vi "Waveform generation_dual color_plane by plane - backupCopy.vi"(0 "Number of Steps":dbl, 1 "488 LASER Intensity":dbl(slide) scale=0.0..10.0, 2 "SPIMA Obj Ampl":dbl, 3 "SPIMB Z- galvo amplitude":dbl, 4 "SPIMA Z-Galvo Offset":dbl(slide) scale=0.0..10.0, 5 "SPIMA Z-Galvo Amplitude":dbl(slide) scale=0.0..10.0, 6 "SPIMA Camera trigger":dbl, 7 "SPIMA Obejective Offset":dbl(slide) scale=0.0..10.0, 8 "SPIMB Obejective Offset":dbl(slide) scale=0.0..10.0, 9 "SPIMA Y-Galvo Offset":dbl(slide) scale=0.0..10.0, 10 "SPIMB Camera Trigger":dbl, 11 "561 Laser Amplitude":dbl, 14 "SPIMB Objective Amplitude":dbl(slide) scale=0.0..10.0, 15 "SPIMA Y-Galvo Amplitude":dbl(slide) scale=0.0..10.0, 21 "SPIMB Z-offset":dbl, 24 "SPIMB Y Offset":dbl, 25 "SPIMB Y Amplitude":dbl) -> (20 "DAQ 2":waveform(dbl)[](array[waveform]), 27 "DAQ1":waveform(dbl)[](array[waveform]))   [LabVIEW 2016]
uses:
  <vilib>/measure/NI_MABase.lvlib
panel:
  out "Numeric":i32
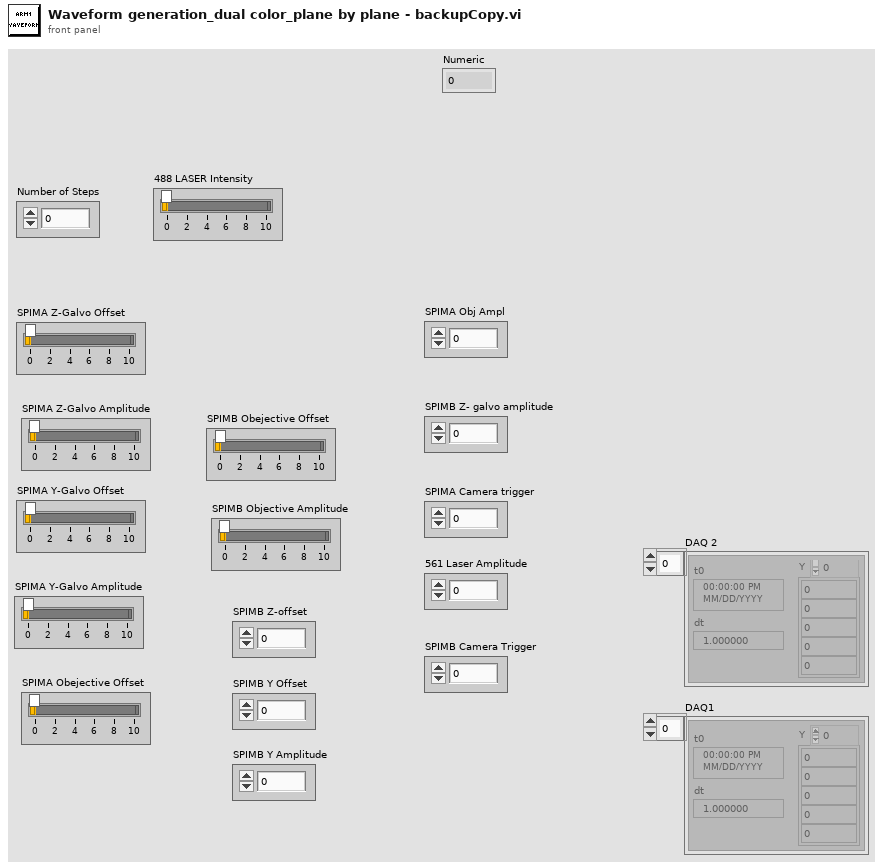
[diagram p1: front panel]
types:
  T1 = enum16{"Sine Wave", "Triangle Wave", "Square Wave", "Sawtooth Wave"}
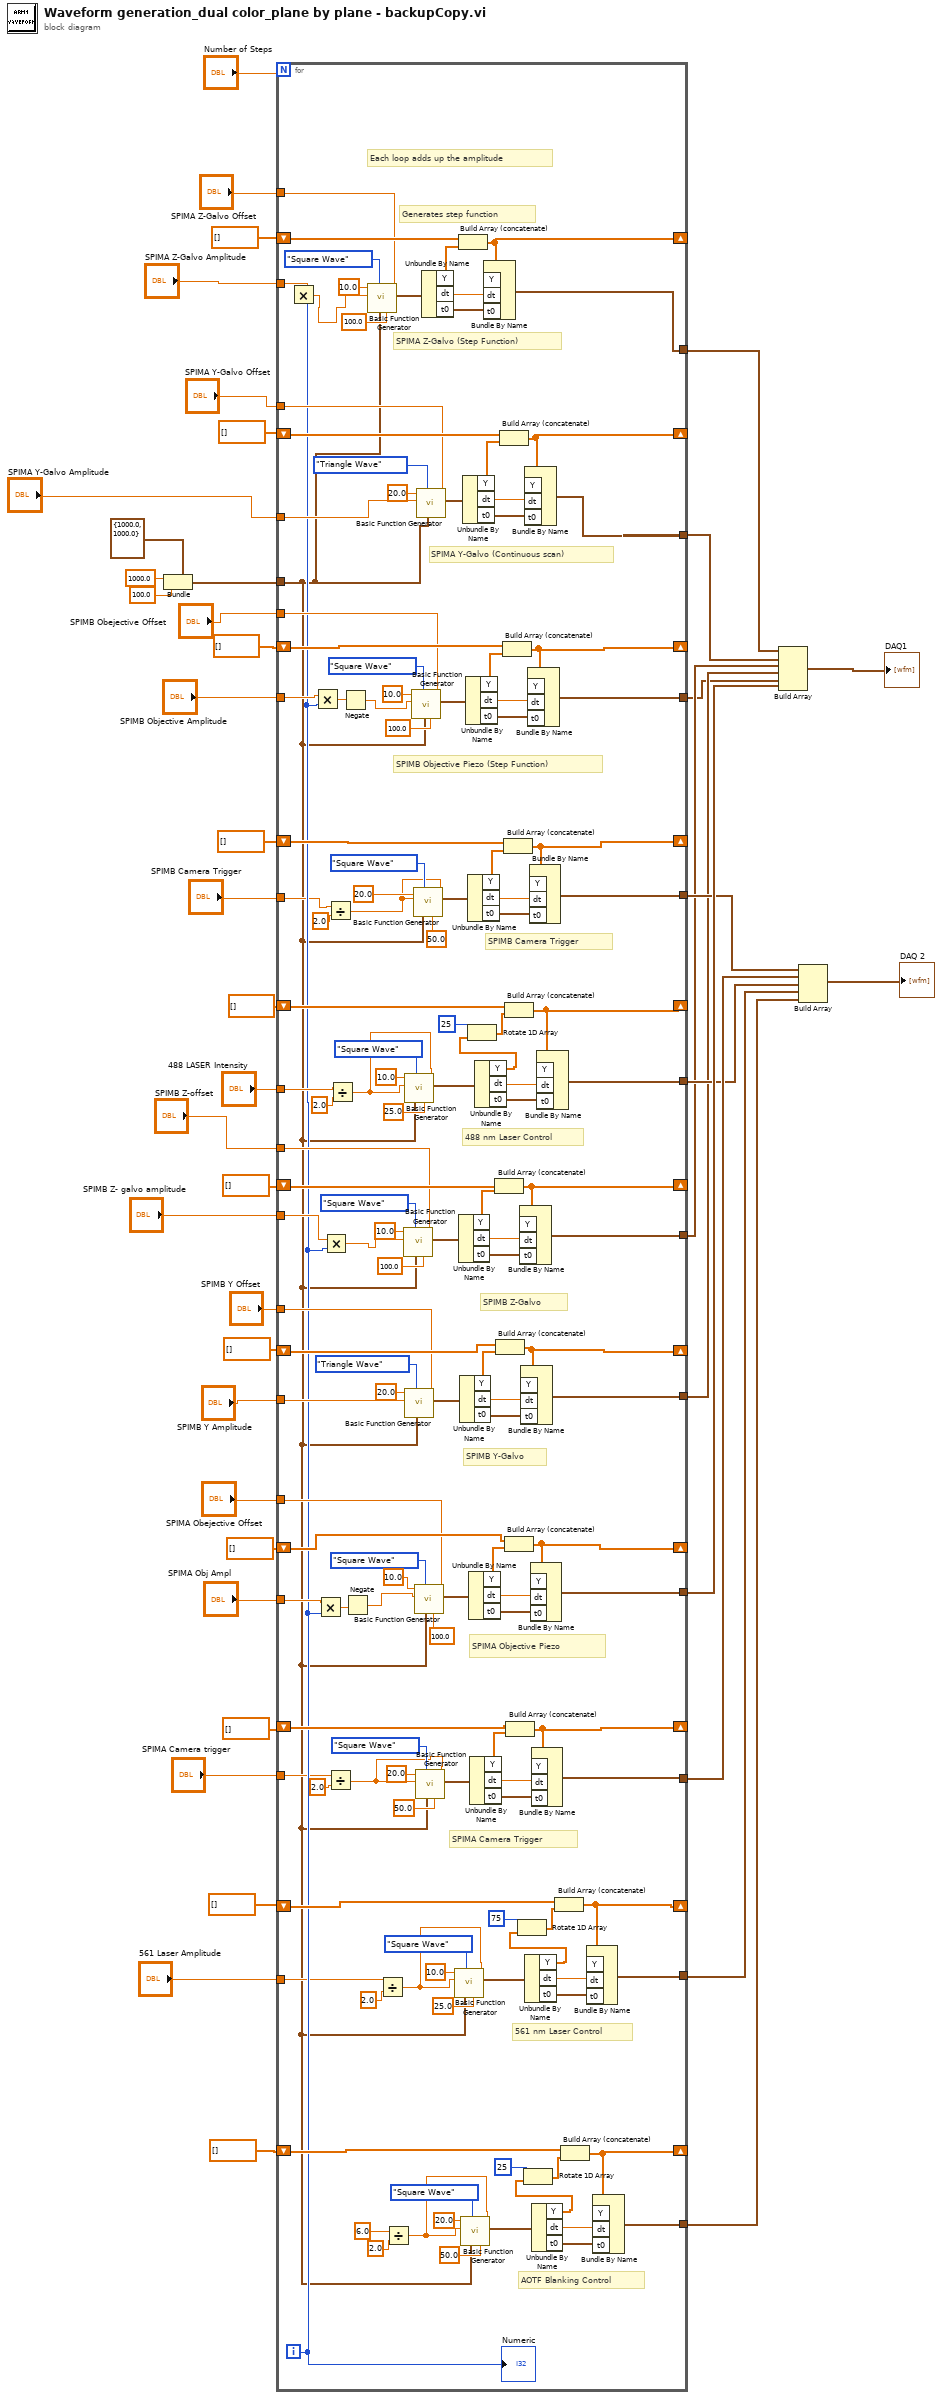
[diagram p0: block diagram]
diagram:
  n1 = Bundle(cluster=cluster{"Fs":dbl, "#s":dbl} {"Fs"=1000.0, "#s"=1000.0} ("sampling info"), "Fs"=1000.0, "#s"=100.0) -> (w42:cluster{"Fs":dbl, "#s":dbl})
  n2 = for {
    N: "Number of Steps" -> [_]
    shift-right: [w186] -> _
    shift-left: dbl[] [] ("appended array") -> [w187]
    tunnel: [w185] -> w34
    shift-right: [w179] -> _
    shift-left: dbl[] [] ("appended array") -> [w180]
    tunnel: [w178] -> w25
    tunnel: w42 -> [w49]
    shift-right: [w153] -> _
    shift-left: dbl[] [] ("appended array") -> [w154]
    tunnel: [w152] -> w16
    shift-right: [w150] -> _
    shift-left: dbl[] [] ("appended array") -> [w151]
    tunnel: [w149] -> w24
    tunnel: "SPIMA Z-Galvo Offset" -> [w148]
    tunnel: "SPIMA Y-Galvo Offset" -> [w147]
    tunnel: "SPIMB Obejective Offset" -> [w146]
    tunnel: "488 LASER Intensity" -> [w98]
    tunnel: [w125] -> w18
    tunnel: [w124] -> w17
    tunnel: [w123] -> w33
    tunnel: [w122] -> w32
    shift-right: [w120] -> _
    shift-left: dbl[] [] ("appended array") -> [w121]
    shift-right: [w118] -> _
    shift-left: dbl[] [] ("appended array") -> [w119]
    shift-right: [w116] -> _
    shift-left: dbl[] [] ("appended array") -> [w117]
    shift-right: [w114] -> _
    shift-left: dbl[] [] ("appended array") -> [w115]
    tunnel: "SPIMA Z-Galvo Amplitude" -> [w113]
    tunnel: "SPIMB Objective Amplitude" -> [w111]
    tunnel: "SPIMA Y-Galvo Amplitude" -> [w109]
    tunnel: "SPIMA Obejective Offset" -> [w108]
    shift-right: [w102] -> _
    shift-left: dbl[] [] ("appended array") -> [w105]
    tunnel: [w106] -> w20
    tunnel: "SPIMB Z-offset" -> [w95]
    tunnel: "SPIMB Y Offset" -> [w94]
    tunnel: "SPIMB Y Amplitude" -> [w93]
    shift-right: [w66] -> _
    shift-left: dbl[] [] ("appended array") -> [w67]
    shift-right: [w64] -> _
    shift-left: dbl[] [] ("appended array") -> [w65]
    tunnel: [w63] -> w9
    tunnel: [w62] -> w8
    tunnel: "SPIMB Z- galvo amplitude" -> [w61]
    tunnel: "SPIMA Obj Ampl" -> [w60]
    tunnel: "SPIMA Camera trigger" -> [w56]
    tunnel: "561 Laser Amplitude" -> [w53]
    tunnel: "SPIMB Camera Trigger" -> [w52]
    i -> [w59]
    # "AOTF Blanking Control"
    # "561 nm Laser Control"
    # "Each loop adds up the amplitude"
    # "Generates step function"
    # "SPIMA Camera Trigger"
    # "SPIMA Objective Piezo"
    # "SPIMB Y-Galvo"
    # "SPIMB Z-Galvo"
    # "488 nm Laser Control"
    # "SPIMB Camera Trigger"
    # "SPIMB Objective Piezo (Step Function)"
    # "SPIMA Y-Galvo (Continuous scan)"
    # "SPIMA Z-Galvo (Step Function)"
    n3 = Multiply(x=w113, y=w59) -> (x*y=w47:dbl)
    n4 = Multiply(x=w111, y=w59) -> (x*y=w112:dbl)
    n5 = Multiply(x=w60, y=w59) -> (x*y=w58:dbl)
    n6 = Multiply(x=w61, y=w59) -> (x*y=w46:dbl)
    n7 = Divide(x=w52, y=2.0) -> (x/y=w50:dbl)
    n8 = Divide(x=w56, y=2.0) -> (x/y=w54:dbl)
    n9 = Divide(x=w98, y=2.0) -> (x/y=w96:dbl)
    n10 = Negate(x=w112) -> (-x=w110:dbl)
    n11 = Negate(x=w58) -> (-x=w57:dbl)
    n12 = call <vilib>:"Basic Function Generator.vi"("offset"=w148, "square wave duty cycle (%)"=100.0, "sampling info"=w49, "signal type"=T1."Square Wave", "amplitude"=w47, "frequency"=10.0) -> ("signal out"=w188:waveform(dbl))  [unwired: 3 in, 2 out]
    n13 = Divide(x=w53, y=2.0) -> (x/y=w82:dbl)
    n14 = Divide(x=6.0, y=2.0) -> (x/y=w71:dbl)
    n15 = call <vilib>:"Basic Function Generator.vi"("offset"=w95, "square wave duty cycle (%)"=100.0, "sampling info"=w49, "signal type"=T1."Square Wave", "amplitude"=w46, "frequency"=10.0) -> ("signal out"=w157:waveform(dbl))  [unwired: 3 in, 2 out]
    n16 = call <vilib>:"Basic Function Generator.vi"("offset"=w96, "square wave duty cycle (%)"=25.0, "sampling info"=w49, "signal type"=T1."Square Wave", "amplitude"=w96, "frequency"=10.0) -> ("signal out"=w107:waveform(dbl))  [unwired: 3 in, 2 out]
    n17 = call <vilib>:"Basic Function Generator.vi"("offset"=w94, "sampling info"=w49, "signal type"=T1."Triangle Wave", "amplitude"=w93, "frequency"=20.0) -> ("signal out"=w142:waveform(dbl))  [unwired: 4 in, 2 out]
    n18 = call <vilib>:"Basic Function Generator.vi"("offset"=w146, "square wave duty cycle (%)"=100.0, "sampling info"=w49, "signal type"=T1."Square Wave", "amplitude"=w110, "frequency"=10.0) -> ("signal out"=w171:waveform(dbl))  [unwired: 3 in, 2 out]
    n19 = call <vilib>:"Basic Function Generator.vi"("offset"=w50, "square wave duty cycle (%)"=50.0, "sampling info"=w49, "signal type"=T1."Square Wave", "amplitude"=w50, "frequency"=20.0) -> ("signal out"=w165:waveform(dbl))  [unwired: 3 in, 2 out]
    n20 = call <vilib>:"Basic Function Generator.vi"("offset"=w108, "square wave duty cycle (%)"=100.0, "sampling info"=w49, "signal type"=T1."Square Wave", "amplitude"=w57, "frequency"=10.0) -> ("signal out"=w135:waveform(dbl))  [unwired: 3 in, 2 out]
    n21 = call <vilib>:"Basic Function Generator.vi"("offset"=w54, "square wave duty cycle (%)"=50.0, "sampling info"=w49, "signal type"=T1."Square Wave", "amplitude"=w54, "frequency"=20.0) -> ("signal out"=w128:waveform(dbl))  [unwired: 3 in, 2 out]
    n22 = call <vilib>:"Basic Function Generator.vi"("offset"=w147, "sampling info"=w49, "signal type"=T1."Triangle Wave", "amplitude"=w109, "frequency"=20.0) -> ("signal out"=w181:waveform(dbl))  [unwired: 4 in, 2 out]
    n23 = Unbundle By Name(w188) -> ("Y"=w189:dbl[], "dt"=w176:dbl, "t0"=w177:timestamp)
    n24 = call <vilib>:"Basic Function Generator.vi"("offset"=w82, "square wave duty cycle (%)"=25.0, "sampling info"=w49, "signal type"=T1."Square Wave", "amplitude"=w82, "frequency"=10.0) -> ("signal out"=w88:waveform(dbl))  [unwired: 3 in, 2 out]
    n25 = Build Array (concatenate)(w187, w189) -> (w186:dbl[])
    n26 = Unbundle By Name(w157) -> ("Y"=w158:dbl[], "dt"=w155:dbl, "t0"=w156:timestamp)
    n27 = Unbundle By Name(w142) -> ("Y"=w143:dbl[], "dt"=w140:dbl, "t0"=w141:timestamp)
    n28 = call <vilib>:"Basic Function Generator.vi"("offset"=w71, "square wave duty cycle (%)"=50.0, "sampling info"=w49, "signal type"=T1."Square Wave", "amplitude"=w71, "frequency"=20.0) -> ("signal out"=w77:waveform(dbl))  [unwired: 3 in, 2 out]
    n29 = Unbundle By Name(w181) -> ("Y"=w182:dbl[], "dt"=w183:dbl, "t0"=w184:timestamp)
    n30 = Unbundle By Name(w171) -> ("Y"=w172:dbl[], "dt"=w169:dbl, "t0"=w170:timestamp)
    n31 = Unbundle By Name(w165) -> ("Y"=w166:dbl[], "dt"=w163:dbl, "t0"=w164:timestamp)
    n32 = Unbundle By Name(w135) -> ("Y"=w136:dbl[], "dt"=w133:dbl, "t0"=w134:timestamp)
    n33 = Unbundle By Name(w128) -> ("Y"=w129:dbl[], "dt"=w126:dbl, "t0"=w127:timestamp)
    n34 = Unbundle By Name(w107) -> ("Y"=w90:dbl[], "dt"=w104:dbl, "t0"=w103:timestamp)
    n35 = Rotate 1D Array(1:w90, 2:25 ("n")) -> (0:w91:dbl[])
    n36 = Bundle By Name("Y"=w186, "dt"=w176, "t0"=w177) -> (w185:waveform(dbl))  [unwired: 1 in]
    n37 = Build Array (concatenate)(w121, w158) -> (w120:dbl[])
    n38 = Build Array (concatenate)(w119, w143) -> (w118:dbl[])
    n39 = Build Array (concatenate)(w180, w182) -> (w179:dbl[])
    n40 = Build Array (concatenate)(w154, w172) -> (w153:dbl[])
    n41 = Build Array (concatenate)(w151, w166) -> (w150:dbl[])
    n42 = Build Array (concatenate)(w105, w91) -> (w102:dbl[])
    n43 = Build Array (concatenate)(w117, w136) -> (w116:dbl[])
    n44 = Build Array (concatenate)(w115, w129) -> (w114:dbl[])
    n45 = Bundle By Name("Y"=w120, "dt"=w155, "t0"=w156) -> (w125:waveform(dbl))  [unwired: 1 in]
    n46 = Bundle By Name("Y"=w118, "dt"=w140, "t0"=w141) -> (w124:waveform(dbl))  [unwired: 1 in]
    n47 = Bundle By Name("Y"=w179, "dt"=w183, "t0"=w184) -> (w178:waveform(dbl))  [unwired: 1 in]
    n48 = Unbundle By Name(w88) -> ("Y"=w79:dbl[], "dt"=w87:dbl, "t0"=w86:timestamp)
    n49 = Rotate 1D Array(1:w79, 2:75 ("n")) -> (0:w80:dbl[])
    n50 = Bundle By Name("Y"=w153, "dt"=w169, "t0"=w170) -> (w152:waveform(dbl))  [unwired: 1 in]
    n51 = Bundle By Name("Y"=w150, "dt"=w163, "t0"=w164) -> (w149:waveform(dbl))  [unwired: 1 in]
    n52 = Bundle By Name("Y"=w116, "dt"=w133, "t0"=w134) -> (w123:waveform(dbl))  [unwired: 1 in]
    n53 = Bundle By Name("Y"=w114, "dt"=w126, "t0"=w127) -> (w122:waveform(dbl))  [unwired: 1 in]
    n54 = Unbundle By Name(w77) -> ("Y"=w68:dbl[], "dt"=w76:dbl, "t0"=w75:timestamp)
    n55 = Rotate 1D Array(1:w68, 2:25 ("n")) -> (0:w69:dbl[])
    n56 = Bundle By Name("Y"=w102, "dt"=w104, "t0"=w103) -> (w106:waveform(dbl))  [unwired: 1 in]
    n57 = Build Array (concatenate)(w67, w80) -> (w66:dbl[])
    n58 = Build Array (concatenate)(w65, w69) -> (w64:dbl[])
    n59 = Bundle By Name("Y"=w66, "dt"=w87, "t0"=w86) -> (w63:waveform(dbl))  [unwired: 1 in]
    n60 = Bundle By Name("Y"=w64, "dt"=w76, "t0"=w75) -> (w62:waveform(dbl))  [unwired: 1 in]
    "Numeric" <- w59
  }
  n61 = Build Array(w34, w25, w18, w17, w16, w33) -> (→"DAQ1":waveform(dbl)[])
  n62 = Build Array(w24, w32, w20, w9, w8) -> (→"DAQ 2":waveform(dbl)[])
